vi "example 10 - resolve data.vi"() -> ()   [LabVIEW 2020]
uses:
  ui-testing.lvlib
panel:
  out "Boolean 2D":bool[][](array[boolean])
  out "Boolean 1D":bool[](array[boolean])
  out "Boolean":bool
  in  "String 2D":string[][](array[string])
  in  "String 1D":string[](array[string])
  in  "String":string="Hello World"
  in  "I64 2D Four":i64[][](array[numeric])=[[0, 1], [2, 3]]
  in  "I64 2D One":i64[][](array[numeric])=[[0]]
  in  "I64 2D Col":i64[][](array[numeric])=[[0], [1]]
  in  "I64 2D Row":i64[][](array[numeric])=[[0, 1]]
  in  "CSG 2D":csg[][](array[numeric])=[[1.2+3.0i, 1.2+3.0i]]
  in  "CXT 2D":cxt[][](array[numeric])=[[1.2345+1.0i, 1.2345+1.0i]]
  in  "CDB 2D":cdb[][](array[numeric])=[[1.23+2.0i, 1.23+2.0i]]
  in  "FXP 2D":fxp<+/-,64,32>[][](array[numeric])=[[0.1229999999050051, 0.1229999999050051]]
  in  "SGL 2D":sgl[][](array[numeric])=[[1.2, 1.2]]
  in  "EXT 2D":ext[][](array[numeric])=[[1.2345, 1.2345]]
  in  "U8 2D":u8[][](array[numeric])=[[8, 8]]
  in  "U16 2D":u16[][](array[numeric])=[[16, 16]]
  in  "U32 2D":u32[][](array[numeric])=[[32, 32]]
  in  "U64 2D":u64[][](array[numeric])=[[64, 64]]
  in  "I8 2D":i8[][](array[numeric])=[[-8, -8]]
  in  "I16 2D":i16[][](array[numeric])=[[-16, -16]]
  in  "I32 2D":i32[][](array[numeric])=[[-32, -32]]
  in  "I64 2D":i64[][](array[numeric])=[[-64, -64]]
  in  "DBL 2D":dbl[][](array[numeric])=[[1.23, 1.23]]
  in  "CSG 1D":csg[](array[numeric])=[1.2+3.0i, 1.2+3.0i]
  in  "CXT 1D":cxt[](array[numeric])=[1.2345+1.0i, 1.2345+1.0i]
  in  "CDB 1D":cdb[](array[numeric])=[1.23+2.0i, 1.23+2.0i]
  in  "FXP 1D":fxp<+/-,64,32>[](array[numeric])=[0.1229999999050051, 0.1229999999050051]
  in  "SGL 1D":sgl[](array[numeric])=[1.2, 1.2]
  in  "EXT 1D":ext[](array[numeric])=[1.2345, 1.2345]
  in  "U8 1D":u8[](array[numeric])=[8, 8]
  in  "U16 1D":u16[](array[numeric])=[16, 16]
  in  "U32 1D":u32[](array[numeric])=[32, 32]
  in  "U64 1D":u64[](array[numeric])=[64, 64]
  in  "I8 1D":i8[](array[numeric])=[-8, -8]
  in  "I16 1D":i16[](array[numeric])=[-16, -16]
  in  "I32 1D":i32[](array[numeric])=[-32, -32]
  in  "I64 1D":i64[](array[numeric])=[-64, -64]
  in  "DBL 1D":dbl[](array[numeric])=[1.23, 1.23]
  in  "CSG":csg=1.2+3.0i
  in  "CXT":cxt=1.2345+1.0i
  in  "CDB":cdb=1.23+2.0i
  in  "FXP":fxp<+/-,64,32>=0.1229999999050051
  in  "SGL":sgl=1.2
  in  "EXT":ext=1.2345
  in  "U8":u8=8
  in  "U16":u16=16
  in  "U32":u32=32
  in  "U64":u64=64
  in  "I8":i8=-8
  in  "I16":i16=-16
  in  "I32":i32=-32
  in  "I64":i64=-64
  in  "DBL":dbl=1.23
  out "Plot":i32[](graph)=[0, 1, 2, 3, 4, 5, 6, 7, 8, 9]
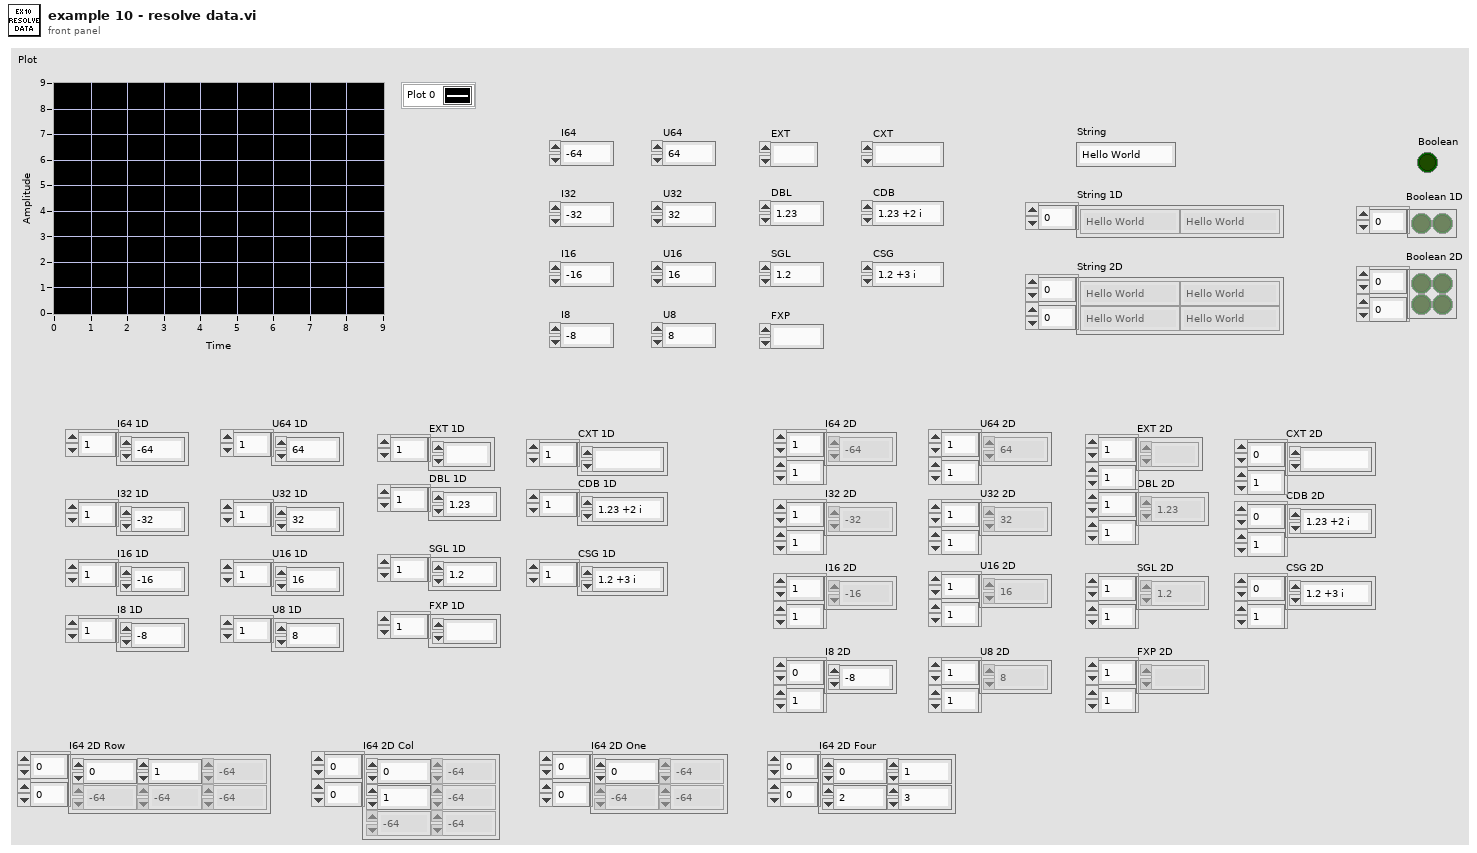
[diagram p1: front panel]
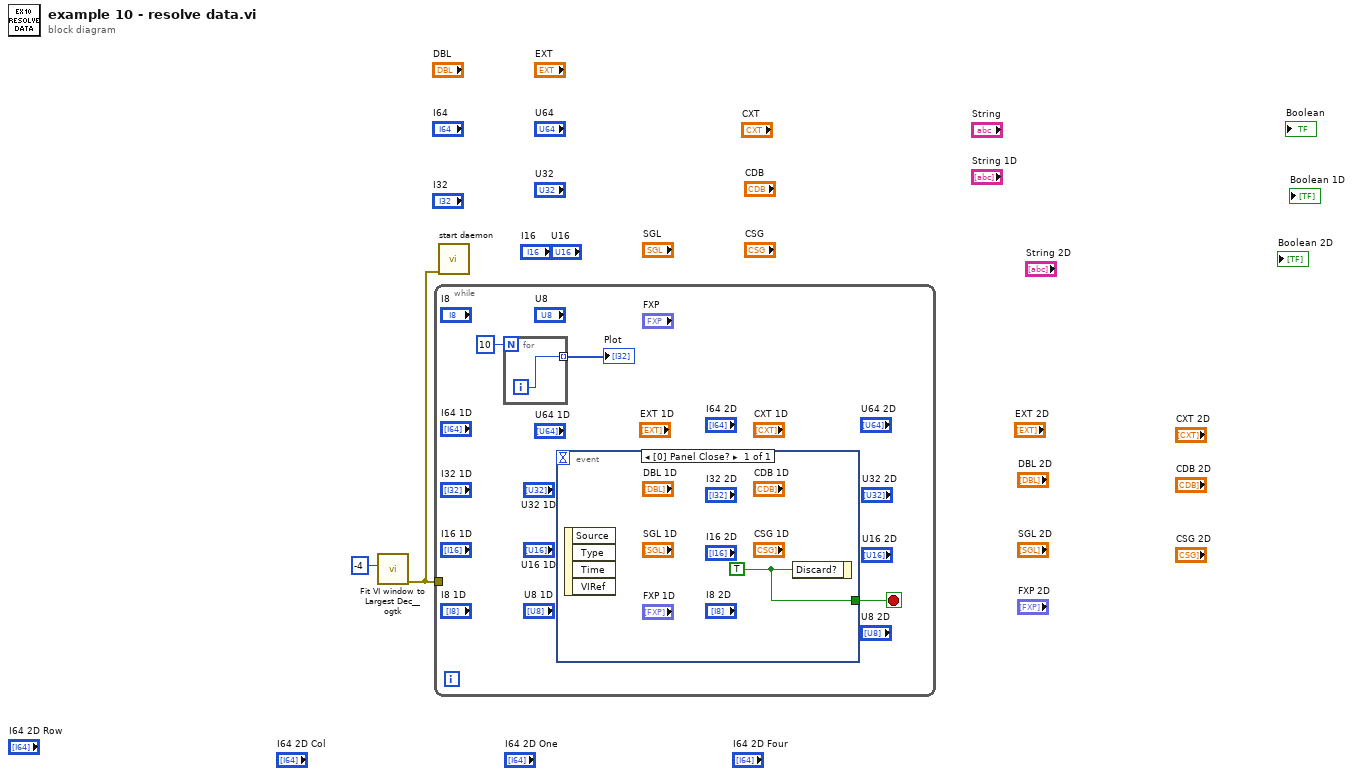
[diagram p0: block diagram]
diagram:
  n1 = call <userlib>:"Fit VI window to Largest Dec__ogtk.vi"("border spacing (2 px)"=-4) -> ("error out"=w1:errorcluster)  [unwired: 5 in, 1 out]
  n2 = while {
    tunnel: w1 -> [_]
    stop <- w5 stop-if-true
    n3 = for {
      N: 10 -> [_]
      tunnel: [w6] -> w4 mode=indexing
      i -> [w6]
    }
    "Plot" <- w4
    n4 = event shown="[0] Panel Close?" {
      selector: _ -> [_]
      dyn-events: _ -> [_]
      timeout: _ -> [_]
      tunnel: [w7] -> w5
      event Panel Close? {
        w7 = TRUE
        n5 = event-data() -> ()  [unwired: 1 in, 4 out]
        n6 = event-data("Discard?"=w7) -> ()  [unwired: 1 in, 1 out]
      }
    }
  }
  n7 = call "start daemon.vi"("error in (no error)"=w1) -> ()  [unwired: 10 in, 1 out]
